vi "From Serial Form.vi"(6 "Serial Version":T1, 10 "Deserializer in":refnum<class "Deserializer.lvclass">=refnum, 11 "Nicholas Data in":refnum<class "Nicholas Data.lvclass">) -> (0 "error out":errorcluster, 2 "Deserializer out":refnum<class "Deserializer.lvclass">, 3 "Nicholas Data out":refnum<class "Nicholas Data.lvclass">)   [LabVIEW 2015, in "Nicholas Data.lvclass"]
uses:
  Nicholas Data.lvclass
  <vilib>/NI/AQ Character Lineator/Serializable/Remove Serializable.vi
  Reusable/CRDS/Data/Main/CRDS Data.lvclass
  Reusable/PAS/Data/Main/PAS Data.lvclass
  Devices/TE Cooler/Data/TECData.lvclass
  Devices/Alicat/Session Based/Data/Alicat Data.lvclass
  Reusable/Data/Array Data/Single 1-D/Single_Array.lvclass
  <vilib>/NI/AQ Character Lineator/Serializable/Remove Boolean Array.vi
  Reusable/Data/Data.lvclass
  <vilib>/NI/AQ Character Lineator/Serialization Common/Serial Version.ctl
  <vilib>/NI/AQ Character Lineator/Deserializer/Deserializer.lvclass
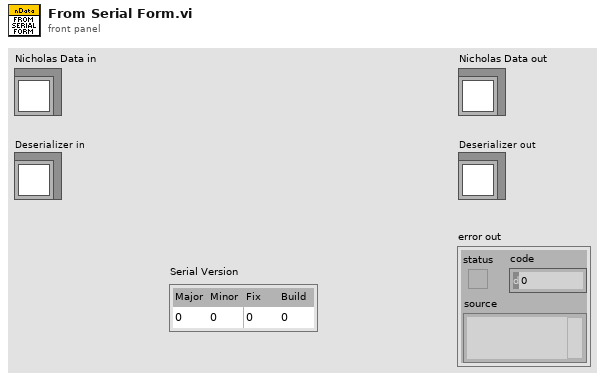
[diagram p1: front panel]
types:
  T1 = typedef "Serialization Common.lvlib/Serial Version.ctl" = cluster{"Major":u16, "Minor":u16, "Fix":u16, "Build":u16}
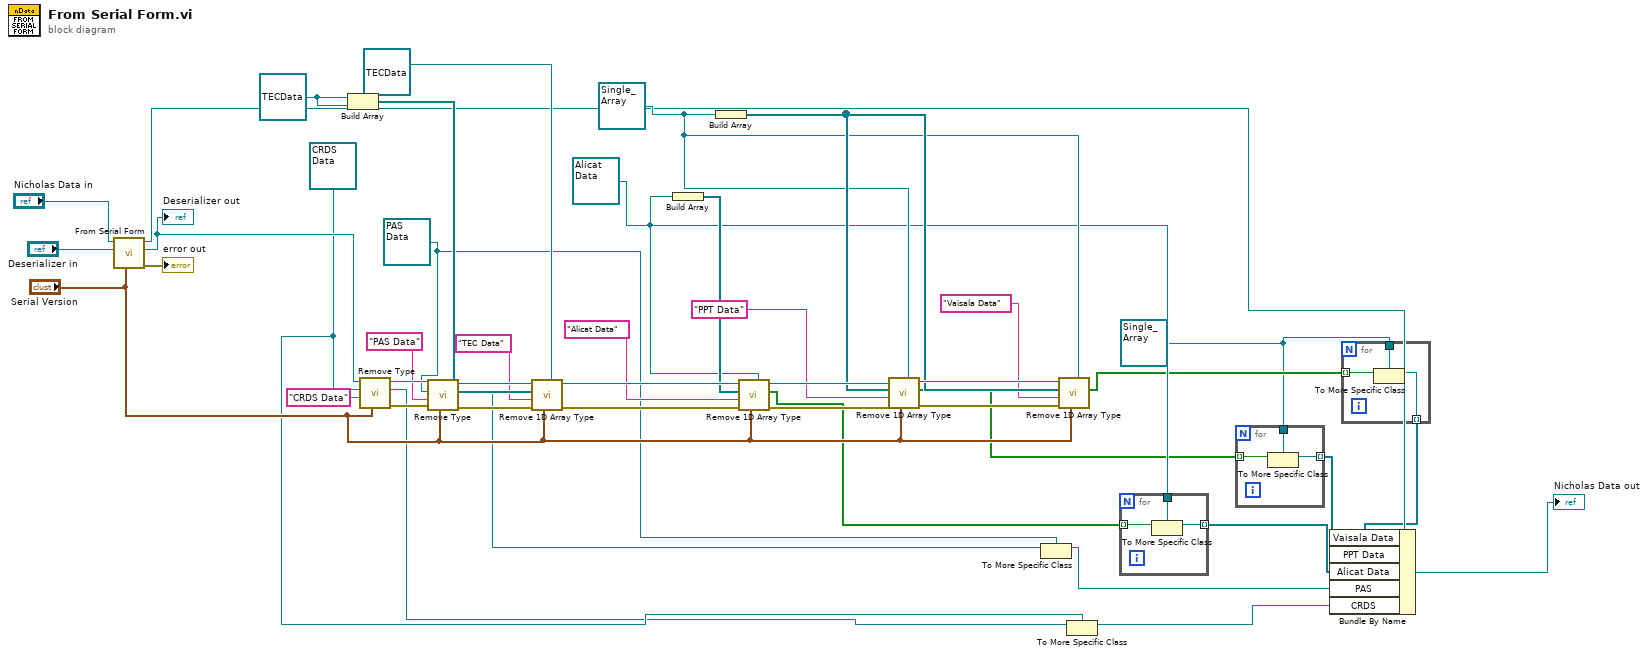
[diagram p0: block diagram]
diagram:
  w3 = refnum<class "Single_Array.lvclass"> refnum ("Base Data Lib:[SGL]")
  w18 = refnum<class "Single_Array.lvclass"> refnum ("Base Data Lib:[SGL]")
  w8 = refnum<class "Alicat Data.lvclass"> refnum ("Alicat Data")
  w34 = refnum<class "TECData.lvclass"> refnum ("TE Cooler.lvlib:TEC Data")
  w11 = refnum<class "PAS Data.lvclass"> refnum ("PAS")
  w15 = refnum<class "CRDS Data.lvclass"> refnum ("CRDS")
  n1 = call-parent "From Serial Form.vi"("Serial Version"="Serial Version", "Deserializer in"="Deserializer in", "Data in"="Nicholas Data in") -> ("error out"=→"error out":errorcluster, "Deserializer out"=w40:refnum<class "Deserializer.lvclass">, "Data out"=w16:refnum<class "Nicholas Data.lvclass">)  [unwired: 6 in]
  "Deserializer out" <- w40
  n2 = Build Array(w34, w34) -> (w33:refnum<class "TECData.lvclass">[])
  n3 = call-poly <vilib>:"Remove Type.vi"("Serial Version"="Serial Version", "Name"="CRDS Data", "Default Value"=w15, "Deserializer in"=w40) -> ("error out"=w37:errorcluster, "Serializable"=w14:refnum<class "Serializable.lvclass">, "Deserializer out"=w38:refnum<class "Deserializer.lvclass">)  [unwired: 4 in, 1 out]
  n4 = call-poly <vilib>:"Remove Type.vi"("Serial Version"="Serial Version", "error in (no error)"=w37, "Name"="PAS Data", "Default Value"=w11, "Deserializer in"=w38) -> ("error out"=w32:errorcluster, "Serializable"=w12:refnum<class "Serializable.lvclass">, "Deserializer out"=w35:refnum<class "Deserializer.lvclass">)  [unwired: 3 in, 1 out]
  n5 = call-poly <vilib>:"Remove 1D Array Type.vi"(5:refnum<class "TECData.lvclass"> refnum ("TE Cooler.lvlib:TEC Data"), 6:"Serial Version", "error in (no error)"=w32, "Name"="TEC Data", "Default Value"=w33, "Deserializer in"=w35) -> ("error out"=w28:errorcluster, "Deserializer out"=w29:refnum<class "Deserializer.lvclass">)  [unwired: 2 in, 2 out]
  n6 = Build Array(w8) -> (w26:refnum<class "Alicat Data.lvclass">[])
  n7 = Build Array(w18) -> (w20:refnum<class "Single_Array.lvclass">[])
  n8 = call-poly <vilib>:"Remove 1D Array Type.vi"(5:w8, 6:"Serial Version", "error in (no error)"=w28, "Name"="Alicat Data", "Default Value"=w26, "Deserializer in"=w29) -> ("error out"=w24:errorcluster, "Booleans"=w9:bool[], "Deserializer out"=w25:refnum<class "Deserializer.lvclass">)  [unwired: 2 in, 1 out]
  n9 = call-poly <vilib>:"Remove 1D Array Type.vi"(5:w18, 6:"Serial Version", "error in (no error)"=w24, "Name"="PPT Data", "Default Value"=w20, "Deserializer in"=w25) -> ("error out"=w21:errorcluster, "Booleans"=w6:bool[], "Deserializer out"=w22:refnum<class "Deserializer.lvclass">)  [unwired: 2 in, 1 out]
  n10 = To More Specific Class(target class=w11, reference=w12) -> (specific class reference=w10:refnum<class "PAS Data.lvclass">)  [unwired: 1 in, 1 out]
  n11 = call-poly <vilib>:"Remove 1D Array Type.vi"(5:w18, 6:"Serial Version", "error in (no error)"=w21, "Name"="Vaisala Data", "Default Value"=w20, "Deserializer in"=w22) -> ("Booleans"=w4:bool[])  [unwired: 2 in, 3 out]
  n12 = To More Specific Class(target class=w15, reference=w14) -> (specific class reference=w13:refnum<class "CRDS Data.lvclass">)  [unwired: 1 in, 1 out]
  n13 = for {
    tunnel: w9 -> [w46] mode=indexing
    tunnel: w8 -> [w45]
    tunnel: [w44] -> w7 mode=indexing
    n14 = To More Specific Class(target class=w45, reference=w46) -> (specific class reference=w44:refnum<class "Alicat Data.lvclass">)  [unwired: 1 in, 1 out]
  }
  n15 = for {
    tunnel: w6 -> [w49] mode=indexing
    tunnel: w3 -> [w48]
    tunnel: [w47] -> w5 mode=indexing
    n16 = To More Specific Class(target class=w48, reference=w49) -> (specific class reference=w47:refnum<class "Single_Array.lvclass">)  [unwired: 1 in, 1 out]
  }
  n17 = for {
    tunnel: w4 -> [w52] mode=indexing
    tunnel: w3 -> [w51]
    tunnel: [w50] -> w2 mode=indexing
    n18 = To More Specific Class(target class=w51, reference=w52) -> (specific class reference=w50:refnum<class "Single_Array.lvclass">)  [unwired: 1 in, 1 out]
  }
  n19 = Bundle By Name(cluster=w16, "Vaisala Data"=w2, "PPT Data"=w5, "Alicat Data"=w7, "PAS"=w10, "CRDS"=w13) -> (→"Nicholas Data out":refnum<class "Nicholas Data.lvclass">)
